vi "Enumerate and Select Camera.vi"() -> ()   [LabVIEW 2023]
doc: "The Enumerate and Select Camera example demonstrates the capability to enumerate the available cameras and dynamically change which camera to acquire from."
uses:
  <vilib>/vision/driver/NI_Vision_Acquisition_Software.lvlib
panel:
  out "Frame Rate":dbl
  out "Buffer Number":u32
  out "Image":T1(plugin-control)
  in  "Stop":bool
  in  "Interfaces":i32(listbox)
  # "Overview: Demonstrates how to enumerate the available cameras, and dynamically change which camera to acquire from.\nRequirements: Vision Acquisition Software, multiple cameras\nInstructions: \n1. Run the VI\n2. Select one of the available Interfaces."
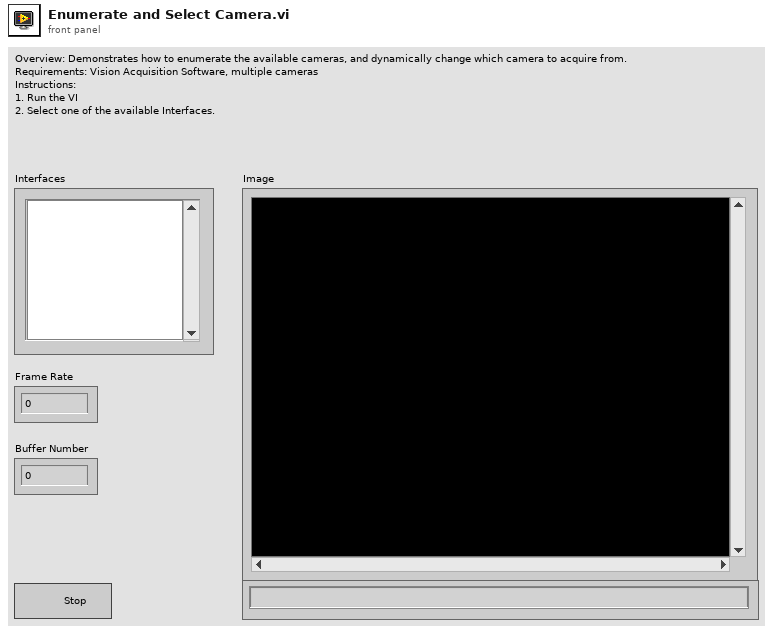
[diagram p1: front panel]
types:
  T1 = typedef "IMAQ Image.ctl" = refnum<image>
  T2 = cluster{"Type":u32, "Version":u32, "Flags":u32, "SerialNumberHigh":u32, "SerialNumberLow":u32, "BusType":u32, "InterfaceName":string, "VendorName":string, "ModelName":string, "CameraFileName":string, "CameraAttributeURL":string}[]
  T3 = typedef "IMAQdx.ctl" = refnum<k21>
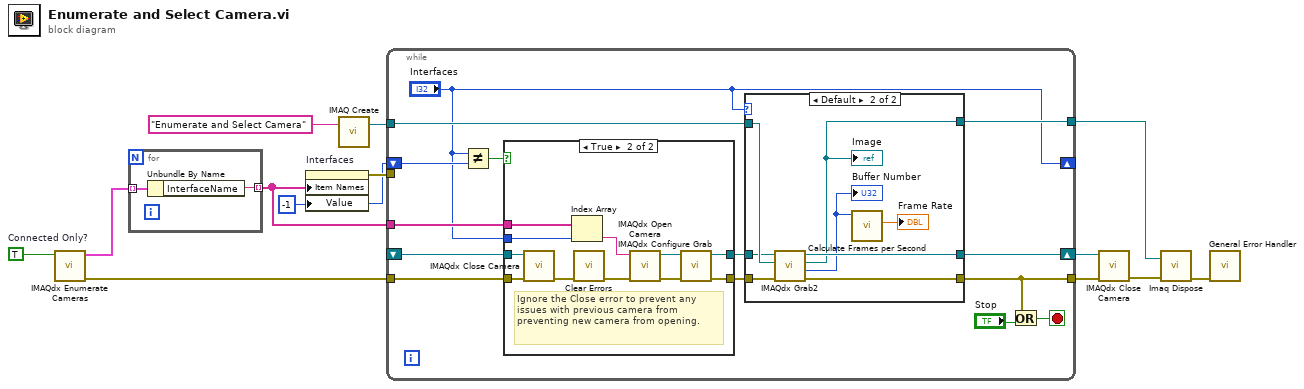
[diagram p0: block diagram]
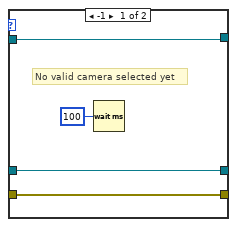
[diagram p2: hidden frame]
diagram:
  w1 = -1 ("Interfaces")
  w6 = TRUE  # Connected Only?
  n1 = call <vilib>:"IMAQdx Enumerate Cameras.vi"("Connected Only? (Yes)"=w6) -> ("error out"=w12:errorcluster, "Camera Information Array"=w7:T2)  [unwired: 1 in, 8 out]
  n2 = for {
    tunnel: w7 -> [w15] mode=indexing
    tunnel: [w14] -> w5 mode=indexing
    n3 = Unbundle By Name(w15) -> ("InterfaceName"=w14:string)
  }
  n4 = property on="Interfaces" class="LstBox (strict)"("Item Names"=w5, "Value"=w1) -> (error out=w8:errorcluster)  [unwired: 2 in, 1 out]
  n5 = call "IMAQ Create"("Image Name"="Enumerate and Select Camera") -> ("New Image"=w10:T1)  [unwired: 3 in, 2 out]
  n6 = while {
    shift-left: w1 -> [w25]
    shift-right: ["Interfaces"] -> _
    tunnel: w10 -> [w28]
    tunnel: w12 -> [w29]
    tunnel: [w19] -> w13
    tunnel: w5 -> [w22]
    shift-right: [w23] -> w9
    shift-left: _ -> [w20]
    tunnel: w8 -> [_]
    tunnel: [w18] -> w4
    stop <- w26 stop-if-true
    n7 = Not Equal?(x="Interfaces", y=w25) -> (x != y?=w17:bool)
    n8 = case shown="True" w17 {
      tunnel: w29 -> [w43 w47]
      tunnel: [w43 w50] -> w24
      tunnel: "Interfaces" -> [_ w54]
      tunnel: w22 -> [_ w53]
      tunnel: [w42 w48] -> w21
      tunnel: w20 -> [w42 w52]
      frame False {
      }
      frame True {
        # "Ignore the Close error to prevent any issues with previous camera from preventing new camera from opening."
        n9 = call <vilib>:"IMAQdx Close Camera.vi"("error in"=w47, "Session In"=w52) -> ("error out"=w45:errorcluster)  [unwired: 9 out]
        n10 = Index Array(array=w53, index=w54) -> (element=w46:string)
        n11 = call <vilib>:"Clear Errors.vi"("error in (no error)"=w45) -> ("error out"=w44:errorcluster)  [unwired: 5 in, 1 out]
        n12 = call <vilib>:"IMAQdx Open Camera.vi"("error in"=w44, "Session In"=w46) -> ("error out"=w51:errorcluster, "Session Out"=w49:T3)  [unwired: 1 in, 7 out]
        n13 = call <vilib>:"IMAQdx Configure Grab.vi"("error in"=w51, "Session In"=w49) -> ("error out"=w50:errorcluster, "Session Out"=w48:T3)  [unwired: 1 in, 7 out]
      }
    }
    n14 = case shown="Default" "Interfaces" {
      tunnel: w28 -> [w33 w41]
      tunnel: w24 -> [w31 w40]
      tunnel: [w32 w39] -> w23
      tunnel: w21 -> [w32 w38]
      tunnel: [w31 w36] -> w19
      tunnel: [w33 w35] -> w18
      frame -1 {
        # "No valid camera selected yet"
        n15 = Wait (ms)(milliseconds to wait=u32 100) -> ()  [unwired: 1 out]
      }
      frame Default {
        n16 = call <vilib>:"IMAQdx Grab2.vi"("error in"=w40, "Image In"=w41, "Session In"=w38) -> ("error out"=w36:errorcluster, "Buffer Number Out"=w37:u32, "Image Out"=w35:T1, "Session Out"=w39:T3)  [unwired: 5 in]
        "Image" <- w35
        "Buffer Number" <- w37
        n17 = call <vilib>:"Calculate Frames per Second.vi"("Buffer Number"=w37) -> ("Processed Frames/s"=→"Frame Rate":dbl)  [unwired: 8 in, 2 out]
      }
    }
    n18 = Or(x=w19, y="Stop") -> (x .or. y?=w26:bool)
  }
  n19 = call <vilib>:"IMAQdx Close Camera.vi"("error in"=w13, "Session In"=w9) -> ("error out"=w3:errorcluster)  [unwired: 9 out]
  n20 = call "Imaq Dispose"("Image"=w4, "error in (no error)"=w3) -> ("error out"=w2:errorcluster)  [unwired: 4 in]
  n21 = call <vilib>:"General Error Handler.vi"("error in (no error)"=w2) -> ()  [unwired: 2 in, 13 out]
